vi "Home All.vi"(8 "error in (no error)":errorcluster, 11 "Gantry in":refnum<class "Gantry.lvclass">) -> (0 "error out":errorcluster, 3 "Gantry out":refnum<class "Gantry.lvclass">)   [LabVIEW 2023, in "Gantry.lvclass"]
uses:
  Gantry.lvclass
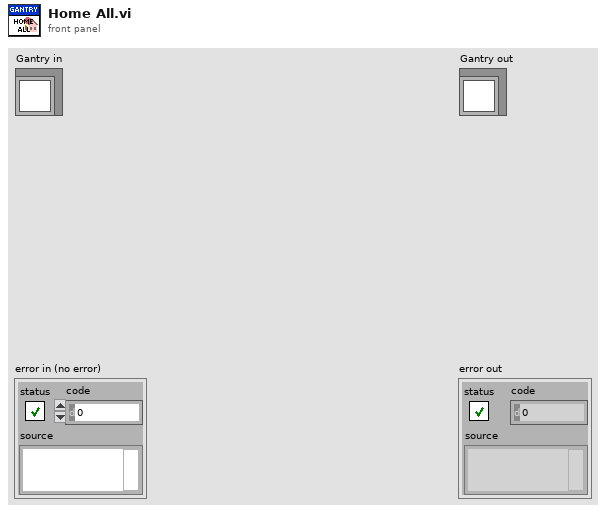
[diagram p1: front panel]
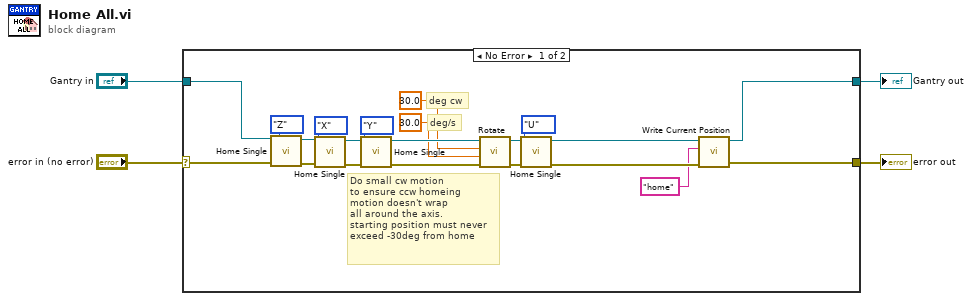
[diagram p0: block diagram]
diagram:
  n1 = case shown="No Error" "error in (no error)" {
    selector: "error in (no error)" -> [w8 w27]
    tunnel: [w7 w27] -> w3
    tunnel: [w6 w26] -> w1
    tunnel: "Gantry in" -> [w5 w26]
    frame No Error {
      # "deg/s"
      # "deg cw"
      # "Do small cw motion\nto ensure ccw homeing\nmotion doesn't wrap \nall around the axis.\nstarting position must never\nexceed -30deg from home"
      n2 = call-dynamic "Home Single.vi"("error in"=w8, "Axis"=enum16{"X", "Y", "Z", "U"}."Z", "Gantry in"=w5) -> ("error out"=w20:errorcluster, "Gantry out"=w22:refnum<class "Gantry.lvclass">)  [unwired: 7 in]
      n3 = call-dynamic "Home Single.vi"("error in"=w20, "Axis"=enum16{"X", "Y", "Z", "U"}."X", "Gantry in"=w22) -> ("error out"=w19:errorcluster, "Gantry out"=w21:refnum<class "Gantry.lvclass">)  [unwired: 7 in]
      n4 = call-dynamic "Home Single.vi"("error in"=w19, "Axis"=enum16{"X", "Y", "Z", "U"}."Y", "Gantry in"=w21) -> ("error out"=w18:errorcluster, "Gantry out"=w17:refnum<class "Gantry.lvclass">)  [unwired: 7 in]
      n5 = call-dynamic "Rotate.vi"("error in"=w18, "speed(deg/s)"=30.0 ("speed"), "distance(deg)"=30.0 ("distance"), "Gantry in"=w17) -> ("error out"=w13:errorcluster, "Gantry out"=w14:refnum<class "Gantry.lvclass">)  [unwired: 6 in]
      n6 = call-dynamic "Home Single.vi"("error in"=w13, "Axis"=enum16{"X", "Y", "Z", "U"}."U", "Gantry in"=w14) -> ("error out"=w24:errorcluster, "Gantry out"=w25:refnum<class "Gantry.lvclass">)  [unwired: 7 in]
      n7 = call-dynamic "Write Current Position.vi"("error in"=w24, "Current Position"="home", "Gantry in"=w25) -> ("error out"=w7:errorcluster, "Gantry out"=w6:refnum<class "Gantry.lvclass">)  [unwired: 7 in]
    }
    frame Error {
    }
  }
  "error out" <- w3
  "Gantry out" <- w1
